vi "Compiled_Settings_to_Settings.vi"(8 "error in (no error)":errorcluster, 11 "Compiled.Settings":T1={"Name"="", "RDB Data Receive "=[], "RDB Data Sent"=[], "vclient"=path "", "Network Settings"={"IP adress"="127.0.0.1", "RDB"={"Protocol"=enum."UDP", "Tx Port"=48190, "Rx Port"=48190, "Buffer Size"=204800, "Timeout"=10}, "SCP"={"Protocol"=enum."UDP", "Tx Port"=0, "Rx Port"=0, "Buffer Size"=204800, "Timeout"=10}}, "SensorInfos"=[], "mmanager"=path "", "Scenario Paths"=[], "Custom SCP Commands"=[], "Timed Loop Settings for TaskControl"={"Period(ms)"=2, "Priority"=100, "Processor"=-2}, "Timed Loop Settings for ModuleManager"={"Period(ms)"=2, "Priority"=100, "Processor"=-2}}) -> (0 "error out":errorcluster, 3 "Settings":T14={"UDP Receiver"=refnum, "UDP Sender"=refnum, "Valid Packet"=FALSE, "TCP"=refnum, "Network Settings"={"IP adress"="", "RDB"={"Protocol"=enum."UDP", "Tx Port"=0, "Rx Port"=0, "Buffer Size"=204800, "Timeout"=10}, "SCP"={"Protocol"=enum."TCP", "Tx Port"=48191, "Rx Port"=48191, "Buffer Size"=204800, "Timeout"=10}}, "vclient"=path "", "paeseHandle"=0})   [LabVIEW 2023]
uses:
  Engine/Type/Settings.ctl
  Shared/Network Settings.ctl
  Shared/Protocol.ctl
  Shared/Compiled.Settings.ctl
  System Explorer/RDB Data.ctl
  RDB/RDB Object.ctl
  RDB/RDB Player Object.ctl
  Shared/SensorInfos.ctl
  Shared/SensorInfo.ctl
  Shared/Sensor Name.ctl
  MM/MM Data.ctl
  MM/MM Objects.ctl
  MM/MM Object.ctl
  Shared/Timedloop Settings.ctl
  Shared/Vires VTD Shared.lvlib
  Engine/Vires VTD Engine.lvlib
  RDB/RDB.lvlib
  MM/MM.lvlib
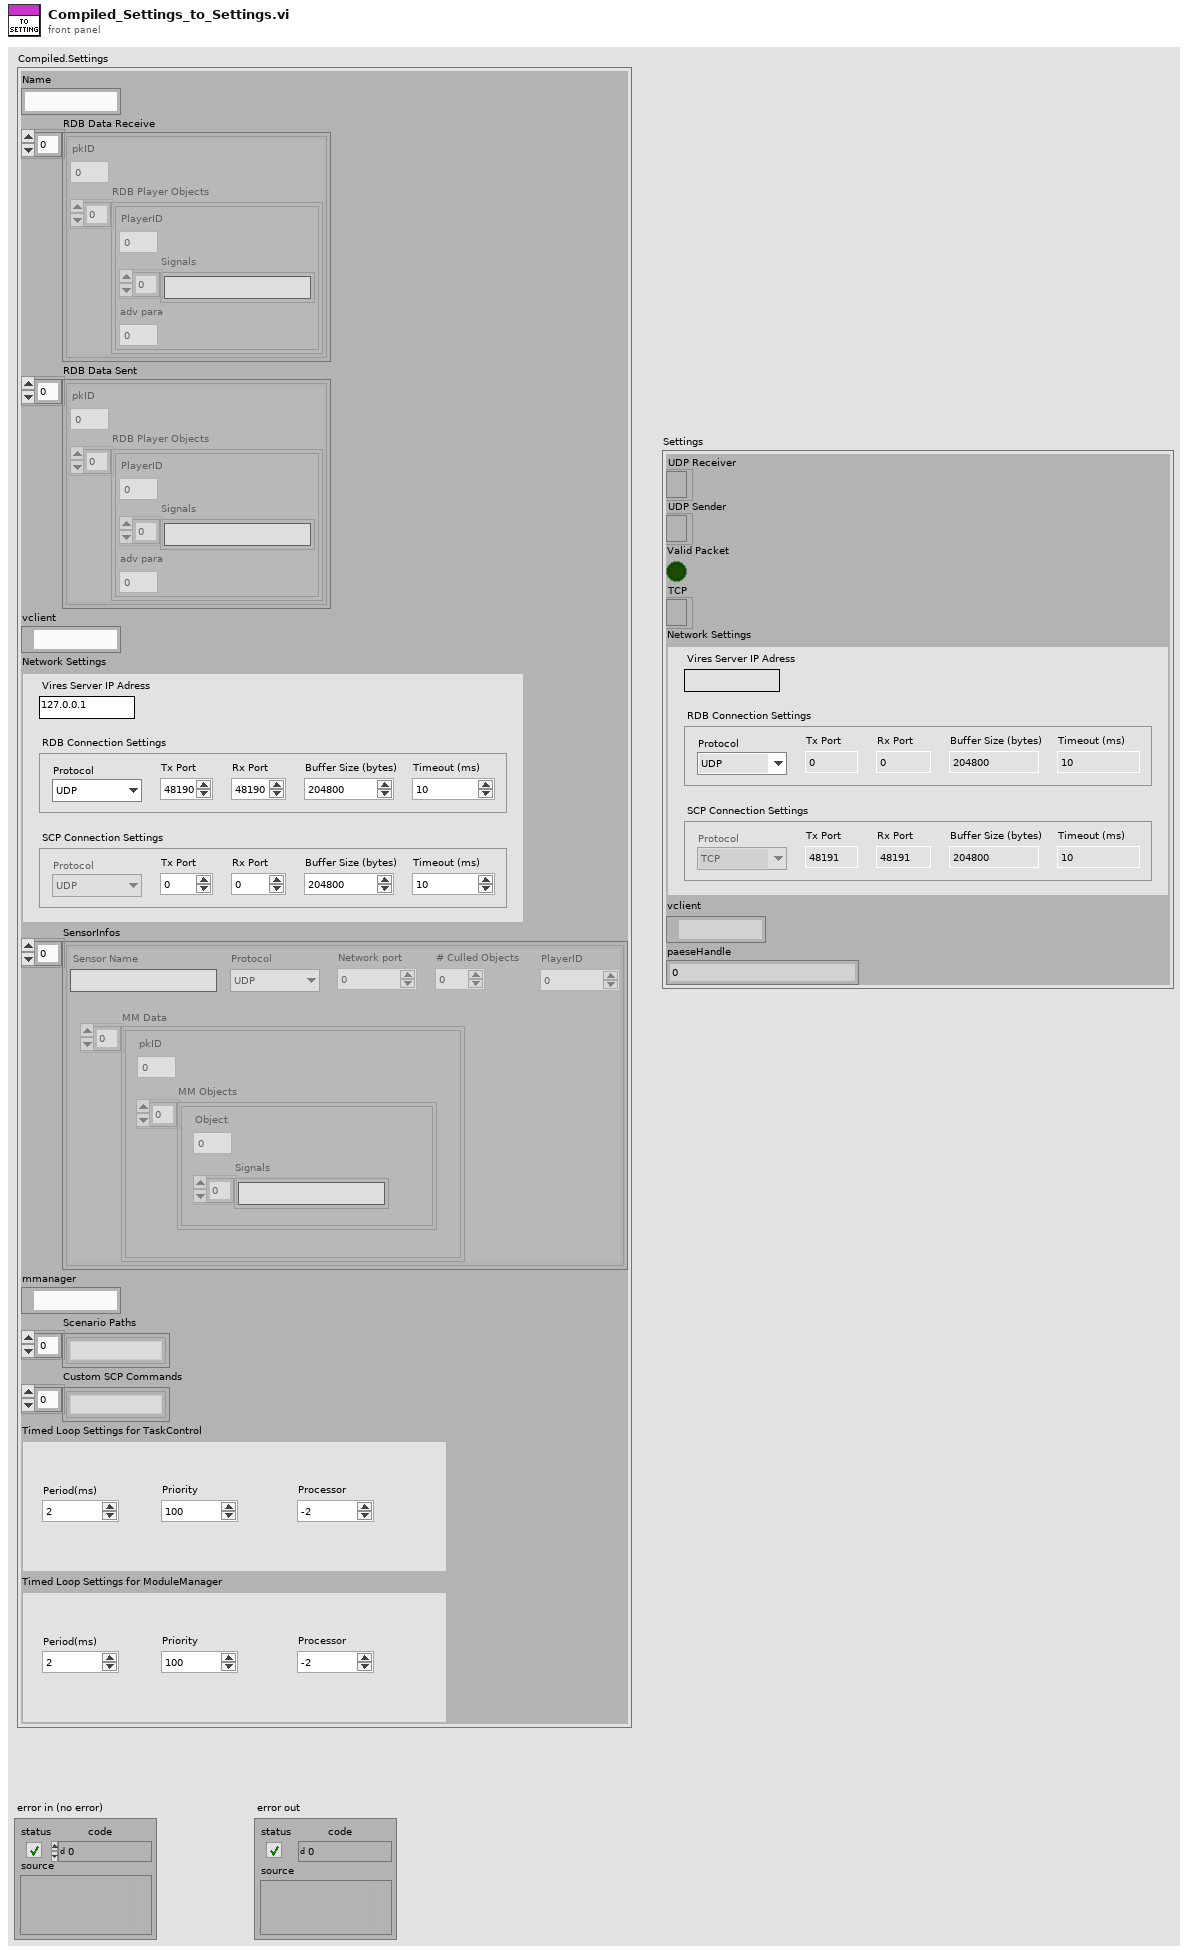
[diagram p1: front panel]
types:
  T1 = typedef "Vires VTD Shared.lvlib/Compiled.Settings.ctl" = cluster{"Name":string, "RDB Data Receive ":T2, "RDB Data Sent":T2, "vclient":path, "Network Settings":T5, "SensorInfos":T7, "mmanager":path, "Scenario Paths":string[], "Custom SCP Commands":string[], "Timed Loop Settings for TaskControl":T13, "Timed Loop Settings for ModuleManager":T13}
  T2 = typedef "Vires VTD Shared.lvlib/RDB Data.ctl" = T3[]
  T3 = typedef "RDB.lvlib/RDB Object.ctl" = cluster{"pkID":i32, "RDB Player Objects":T4[]}
  T4 = typedef "RDB.lvlib/RDB Player Object.ctl" = cluster{"PlayerID":i32, "Signals":string[], "adv para":i32}
  T5 = typedef "Vires VTD Shared.lvlib/Network Settings.ctl" = cluster{"IP adress":string, "RDB":cluster{"Protocol":T6, "Tx Port":u16, "Rx Port":u16, "Buffer Size":i32, "Timeout":u16}, "SCP":cluster{"Protocol":T6, "Tx Port":u16, "Rx Port":u16, "Buffer Size":i32, "Timeout":u16}}
  T6 = typedef "Vires VTD Shared.lvlib/Protocol.ctl" = enum16{"UDP", "TCP"}
  T7 = typedef "Vires VTD Shared.lvlib/SensorInfos.ctl" = T8[]
  T8 = typedef "Vires VTD Shared.lvlib/SensorInfo.ctl" = cluster{"Sensor Name":T9, "Protocol":T6, "Network port":i32, "# Culled Objects":i32, "PlayerID":u8, "MM Data":T10}
  T9 = typedef "Vires VTD Shared.lvlib/Sensor Name.ctl" = string
  T10 = typedef "Vires VTD Shared.lvlib/MM Data.ctl" = T11[]
  T11 = typedef "MM.lvlib/MM Objects.ctl" = cluster{"pkID":i32, "MM Objects":T12[]}
  T12 = typedef "MM.lvlib/MM Object.ctl" = cluster{"Object":i32, "Signals":string[]}
  T13 = typedef "Vires VTD Shared.lvlib/Timedloop Settings.ctl" = cluster{"Period(ms)":i64, "Priority":i32, "Processor":i32}
  T14 = typedef "Vires VTD Engine.lvlib/Settings.ctl" = cluster{"UDP Receiver":refnum<k16>, "UDP Sender":refnum<k16>, "Valid Packet":bool, "TCP":refnum<k5>, "Network Settings":T5, "vclient":path, "paeseHandle":u64}
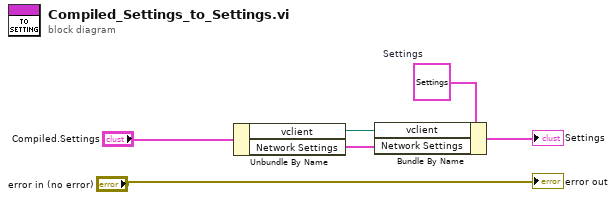
[diagram p0: block diagram]
diagram:
  w3 = T14 {"UDP Receiver"=refnum, "UDP Sender"=refnum, "Valid Packet"=FALSE, "TCP"=refnum, "Network Settings"={"IP adress"="127.0.0.1", "RDB"={"Protocol"=enum."UDP", "Tx Port"=48270, "Rx Port"=10, "Buffer Size"=204800, "Timeout"=10}, "SCP"={"Protocol"=enum."TCP", "Tx Port"=48191, "Rx Port"=48191, "Buffer Size"=204800, "Timeout"=10}}, "vclient"=path "", "paeseHandle"=0}  # Settings
  n1 = Unbundle By Name("Compiled.Settings") -> ("vclient"=w4:path, "Network Settings"=w5:T5)
  n2 = Bundle By Name(cluster=w3, "vclient"=w4, "Network Settings"=w5) -> (→"Settings":T14)
  "error out" <- "error in (no error)"
